vi "serialClose.vi"(8 "error in (no error)":errorcluster, 11 "Python in":T1) -> (0 "error out":errorcluster, 2 "return value":string)   [LabVIEW 2022 SP3]
uses:
  PythonCtrl.ctl
  Processors.ctl
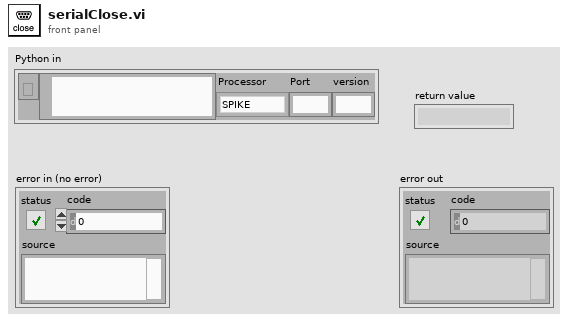
[diagram p1: front panel]
types:
  T1 = typedef "PythonCtrl.ctl" = cluster{"session":refnum<k35>, "PyPath":path, "Processor":T2, "Port":string, "version":string}
  T2 = typedef "Processors.ctl" = enum16{"SPIKE", "Pi", "Pi_ssh", "OpenMV", "Dunio"}
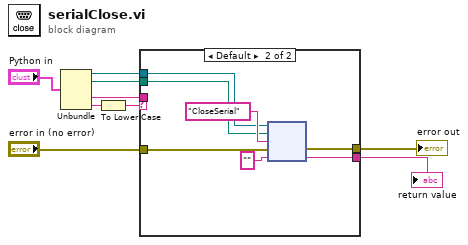
[diagram p0: block diagram]
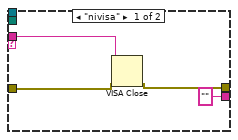
[diagram p2: hidden frame]
diagram:
  n1 = Unbundle("Python in") -> ("session"=w6:refnum<k35>, "PyPath"=w5:path, "Port"=w2:string, "version"=w3:string)  [unwired: 1 out]
  n2 = To Lower Case(string=w3) -> (all lower case string=w1:string)
  n3 = case shown="Default" w1 {
    tunnel: [w11 w20] -> w8
    tunnel: "error in (no error)" -> [w12 w17]
    tunnel: w6 -> [_ w16]
    tunnel: w5 -> [_ w15]
    tunnel: ["" ("function name") w14] -> w4
    tunnel: w2 -> [w13 _]
    frame "nivisa" {
      n4 = VISA Close(VISA resource name=w13, error in (no error)=w12) -> (error out=w11:errorcluster)
    }
    frame Default {
      n5 = node(w16, w15, "CloseSerial" ("function name"), w17, "" ("function name")) -> (w20:errorcluster, w14:string)  [unwired: 3 out]
    }
  }
  "error out" <- w8
  "return value" <- w4
